vi "SetErrorOnVariant.vi"(9 "error info":string, 10 "error code":i32, 11 "body in":variant) -> (3 "body out":variant)   [LabVIEW 2017]
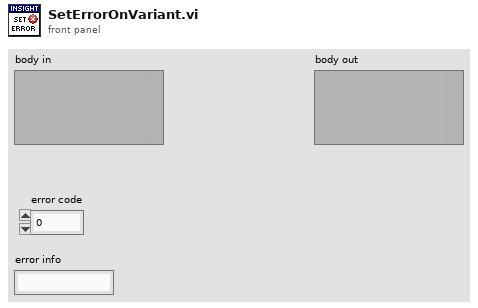
[diagram p1: front panel]
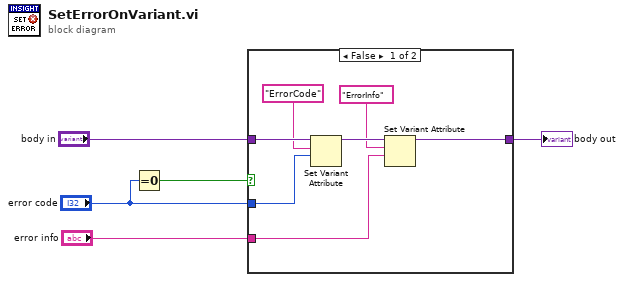
[diagram p0: block diagram]
diagram:
  n1 = Equal To 0?(x="error code") -> (x = 0?=w1:bool)
  n2 = case shown="False" w1 {
    tunnel: "body in" -> [w12 w13]
    tunnel: "error code" -> [w11 _]
    tunnel: "error info" -> [w7 _]
    tunnel: [w6 w13] -> w3
    frame False {
      n3 = Set Variant Attribute(Variant=w12, name="ErrorCode" ("Key"), value=w11) -> (Variant out=w9:variant)  [unwired: 1 in, 2 out]
      n4 = Set Variant Attribute(Variant=w9, name="ErrorInfo" ("Key"), value=w7) -> (Variant out=w6:variant)  [unwired: 1 in, 2 out]
    }
    frame True {
    }
  }
  "body out" <- w3
